vi "Test Config File.vi"() -> ()   [LabVIEW 2025]
doc: "Author: Scott Hannahs <sth@magnet.fsu.edu>\n\nThis software is licensed for use under the “MIT License\"\nCopyright (c) 2025 Scott Hannahs, sth@sth@magnet.sthnet.net\n\nPermission is hereby granted, free of charge, to any person obtaining a copy of this software and associated documentation files (the \"Software\"), to deal in the Software without restriction, including without limitation the rights to use, copy, modify, merge, publish, distribute, sublicense, and/or sell copies of the Software, and to permit persons to whom the Software is furnished to do so, subject to the following conditions: The above copyright notice and this permission notice shall be included in all copies or substantial portions of the Software.\n\nTHE SOFTWARE IS PROVIDED \"AS IS\", WITHOUT WARRANTY OF ANY KIND, EXPRESS OR IMPLIED, INCLUDING BUT NOT LIMITED TO THE WARRANTIES OF MERCHANTABILITY, FITNESS FOR A PARTICULAR PURPOSE AND NONINFRINGEMENT. IN NO EVENT SHALL THE AUTHORS OR COPYRIGHT HOLDERS BE LIABLE FOR ANY CLAIM, DAMAGES OR OTHER LIABILITY, WHETHER IN AN ACTION OF CONTRACT, TORT OR OTHERWISE, ARISING FROM, OUT OF OR IN CONNECTION WITH THE SOFTWARE OR THE USE OR OTHER DEALINGS IN THE SOFTWARE."
panel:
  out "Variant array":variant[](array[variant])
  in  "Coil":enum16{"HTS", "LTS"}(ring)=enum."LTS"
  in  "Config data":variant[](array[variant])
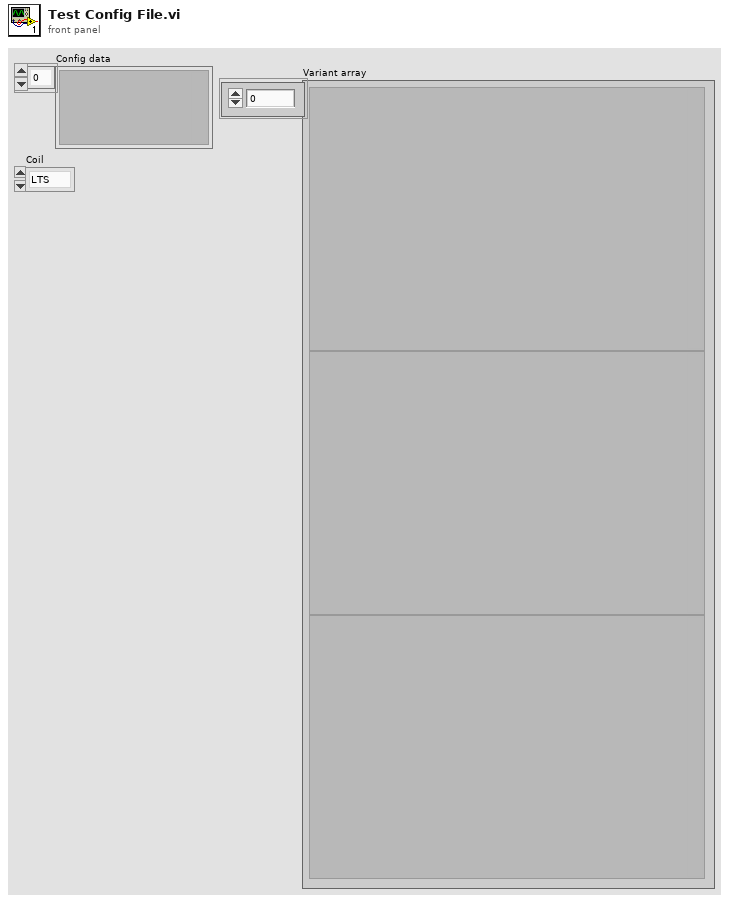
[diagram p1: front panel]
types:
  T1 = typedef "NI_LVConfig.lvlib/Config Data RefNum.ctl" = refnum<k1>
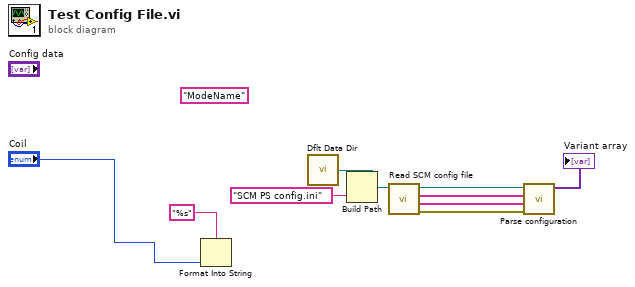
[diagram p0: block diagram]
diagram:
  (unwired) "ModeName"
  n1 = Format Into String(format string="%s", "Coil") -> ()  [unwired: 2 in, 2 out]
  n2 = call <vilib>:"Dflt Data Dir.vi"() -> ("App:Default Data Directory"=w4:path)
  n3 = Build Path(base path=w4, name or relative path="SCM PS config.ini") -> (appended path=w2:path)
  n4 = call "Read SCM config file.vi"("appended path"=w2) -> ("error out"=w5:errorcluster, "Array"=w6:string[], "Array 2"=w7:string[], "Refnum out"=w8:T1)  [unwired: 7 in]
  n5 = call "Parse configuration.vi"("error in (no error)"=w5, "Mode Name for Variant"=w6, "Config File Sections"=w7, "Refnum in"=w8) -> ("Variant array"=→"Variant array":variant[])  [unwired: 6 in, 1 out]
